vi "Sequencer lite.vi"(8 "error in (no error)":errorcluster) -> (0 "Error State":errorcluster)   [LabVIEW 2017]
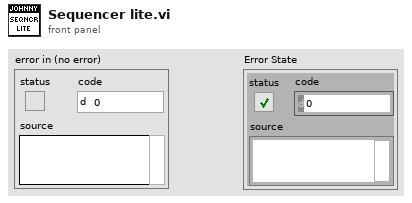
[diagram p1: front panel]
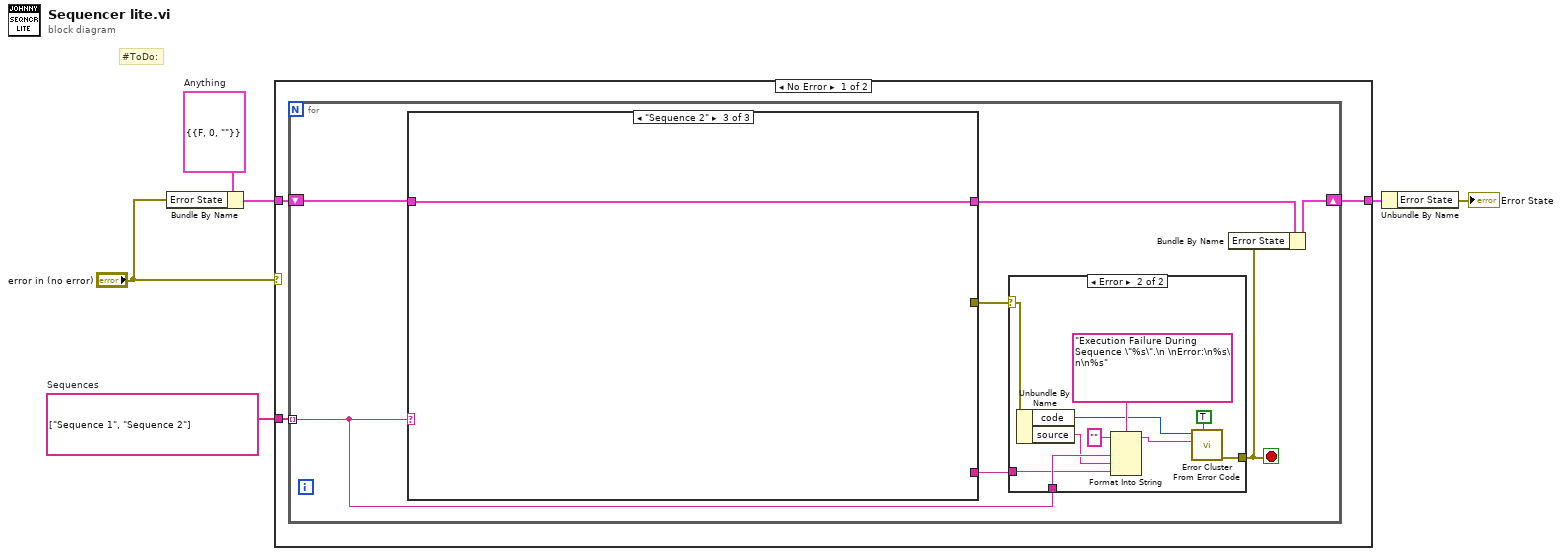
[diagram p0: block diagram]
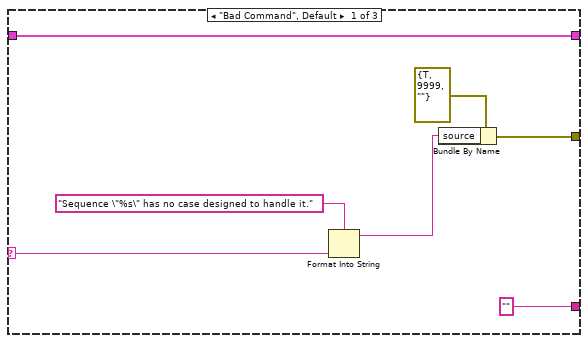
[diagram p3: hidden frame]
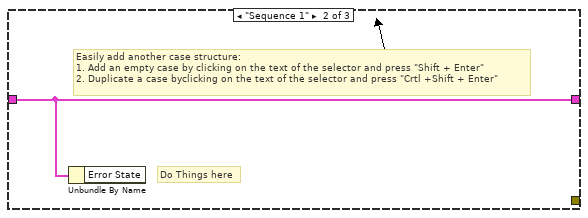
[diagram p4: hidden frame]
diagram:
  w2 = cluster{"Error State":errorcluster} {"Error State"={"status"=FALSE, "code"=0, "source"=""}}  # Anything
  w5 = string[] ["Sequence 1", "Sequence 2"]  # Sequences
  # "#ToDo:"
  n1 = Bundle By Name(cluster=w2, "Error State"="error in (no error)") -> (w6:cluster{"Error State":errorcluster})
  n2 = case shown="No Error" "error in (no error)" {
    tunnel: w5 -> [w9 _]
    tunnel: w6 -> [w8 w37]
    tunnel: [w7 w37] -> w3
    frame No Error {
      n3 = for {
        tunnel: w9 -> [w12] mode=indexing
        shift-right: [w15] -> w7
        shift-left: w8 -> [w16]
        stop <- w10 stop-if-true
        n4 = case shown="\"Sequence 2\"" w12 {
          selector: w12 -> [w29 _ _]
          tunnel: w16 -> [w34 w35 w36]
          tunnel: [w34 w35 w36] -> w14
          tunnel: [w31 _ _] -> w13
          tunnel: ["" ("Accessors:Name") _ _] -> w11
          frame "Bad Command", Default {
            n5 = Format Into String(format string="Sequence \"%s\" has no case designed to handle it.", w29) -> (resulting string=w28:string)  [unwired: 2 in, 1 out]
            n6 = Bundle By Name(cluster=errorcluster {"status"=TRUE, "code"=9999, "source"=""} ("error out"), "source"=w28) -> (w31:errorcluster)
          }
          frame "Sequence 1" {
            # "Easily add another case structure:\n1. Add an empty case by clicking on the text of the selector and press \"Shift + Enter\"\n2. Duplicate a case byclicking on the text of the selector and press \"Crtl +Shift + Enter\""
            # "Do Things here"
            n7 = Unbundle By Name(w35) -> ()  [unwired: 1 out]
          }
          frame "Sequence 2" {
          }
        }
        n8 = case shown="Error" w13 {
          selector: w13 -> [w17 w21]
          tunnel: [w17 w26] -> w10
          tunnel: w12 -> [_ w24]
          tunnel: w11 -> [_ w19]
          frame No Error {
          }
          frame Error {
            n9 = Unbundle By Name(w21) -> ("code"=w18:i32, "source"=w20:string)
            n10 = Format Into String(format string="Execution Failure During Sequence \"%s\".\n \nError:\n%s\n\n%s" ("error message (\"\")"), initial string="", w24, w20, w19) -> (resulting string=w25:string)  [unwired: 1 in, 1 out]
            n11 = call <vilib>:"Error Cluster From Error Code.vi"("show call chain? (False)"=TRUE, "error message (\"\")"=w25, "error code (0)"=w18) -> ("error out"=w26:errorcluster)  [unwired: 6 in]
          }
        }
        n12 = Bundle By Name(cluster=w14, "Error State"=w10) -> (w15:cluster{"Error State":errorcluster})
      }
    }
    frame Error {
    }
  }
  n13 = Unbundle By Name(w3) -> ("Error State"=→"Error State":errorcluster)
